vi "TestPathCommands.vi"(8 "error in (no error)":errorcluster) -> (0 "error out":errorcluster)   [LabVIEW 2019]
uses:
  <vilib>/addons/_JKI Toolkits/Caraya/classes/Test/Test.lvclass
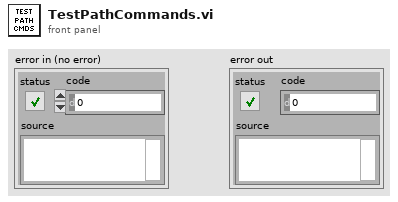
[diagram p1: front panel]
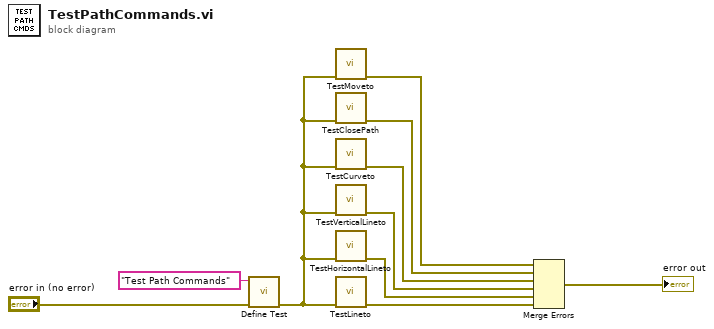
[diagram p0: block diagram]
diagram:
  n1 = call <vilib>:"Define Test.vi"("error in (no error)"="error in (no error)", "Label (VI Title)"="Test Path Commands") -> ("error out"=w2:errorcluster)  [unwired: 8 in, 1 out]
  n2 = call "TestMoveto.vi"("error in (no error)"=w2) -> ("error out"=w10:errorcluster)  [unwired: 10 in]
  n3 = call "TestClosePath.vi"("error in (no error)"=w2) -> ("error out"=w9:errorcluster)  [unwired: 10 in]
  n4 = call "TestCurveto.vi"("error in (no error)"=w2) -> ("error out"=w8:errorcluster)  [unwired: 10 in]
  n5 = call "TestVerticalLineto.vi"("error in (no error)"=w2) -> ("error out"=w7:errorcluster)  [unwired: 10 in]
  n6 = call "TestHorizontalLineto.vi"("error in (no error)"=w2) -> ("error out"=w6:errorcluster)  [unwired: 10 in]
  n7 = call "TestLineto.vi"("error in (no error)"=w2) -> ("error out"=w4:errorcluster)  [unwired: 10 in]
  n8 = Merge Errors(w10, w9, w8, w7, w6, w4) -> (→"error out":errorcluster)
